vi "Create PID Controller.vi"(8 "error in (no error)":errorcluster, 10 "Settings":T3, 11 "Custom Device Ref":refnum<k24>) -> (0 "error out":errorcluster, 3 "Custom Device Ref":refnum<k24>)   [LabVIEW 2013, in "Control SysDef API.lvlib"]
uses:
  Control SysDef API.lvlib
  NationalInstruments.VeriStand.SystemDefinitionAPI
  Shared/Types/Controller Settings.ctl
  Shared/Types/PID Parameters.ctl
  Shared/Types/Action.ctl
  Shared/Constants.vi
  <vilib>/NI Veristand/Custom Device API/NI VeriStand - Set Item Property.vi
  <vilib>/NI Veristand/Custom Device API/Set Item Property (Double).vi
  <vilib>/NI Veristand/Custom Device API/Set Item Property (Boolean).vi
  <vilib>/NI Veristand/Custom Device Tools/Custom Device Utility Library/NI VeriStand - Search for Item.vi
  <vilib>/NI Veristand/Custom Device Tools/Custom Device Utility Library/NI VeriStand - Search for Item by GUID.vi
  <vilib>/NI Veristand/Custom Device API/NI VeriStand - Add Custom Device Channel.vi
  <vilib>/NI Veristand/Custom Device API/NI VeriStand - Remove Custom Device Item.vi
  <vilib>/NI Veristand/Custom Device API/Set Item Property (String).vi
  Shared/Control Addon Shared.lvlib
  <vilib>/NI Veristand/Custom Device API/Custom Device API.lvlib
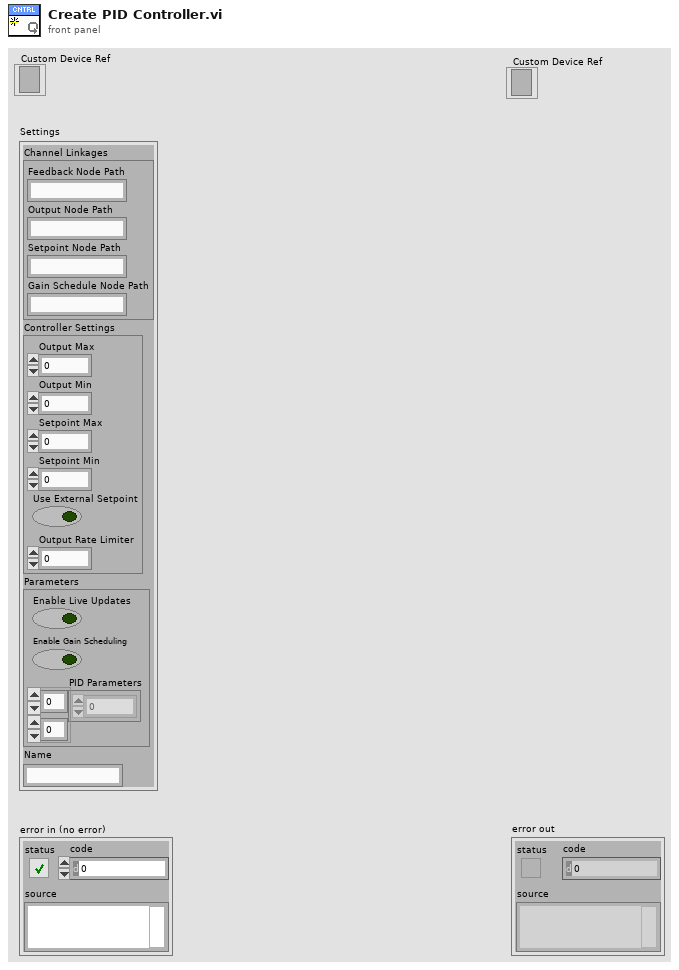
[diagram p1: front panel]
types:
  T1 = typedef "Control Addon Shared.lvlib/Controller Settings.ctl" = cluster{"Output Max":dbl, "Output Min":dbl, "Setpoint Max":dbl, "Setpoint Min":dbl, "Use External Setpoint":bool, "Output Rate Limiter":dbl}
  T2 = typedef "Control Addon Shared.lvlib/PID Parameters.ctl" = cluster{"Enable Live Updates":bool, "Enable Gain Scheduling":bool, "PID Parameters":dbl[][]}
  T3 = cluster{"Channel Linkages":cluster{"Feedback Node Path":string, "Output Node Path":string, "Setpoint Node Path":string, "Gain Schedule Node Path":string}, "Controller Settings":T1, "Parameters":T2, "Name":string}
  T4 = typedef "Control Addon Shared.lvlib/Action.ctl" = enum16{"Get", "Set"}
  T5 = typedef "Custom Device API.lvlib/Custom Device Item Ref.ctl" = u64
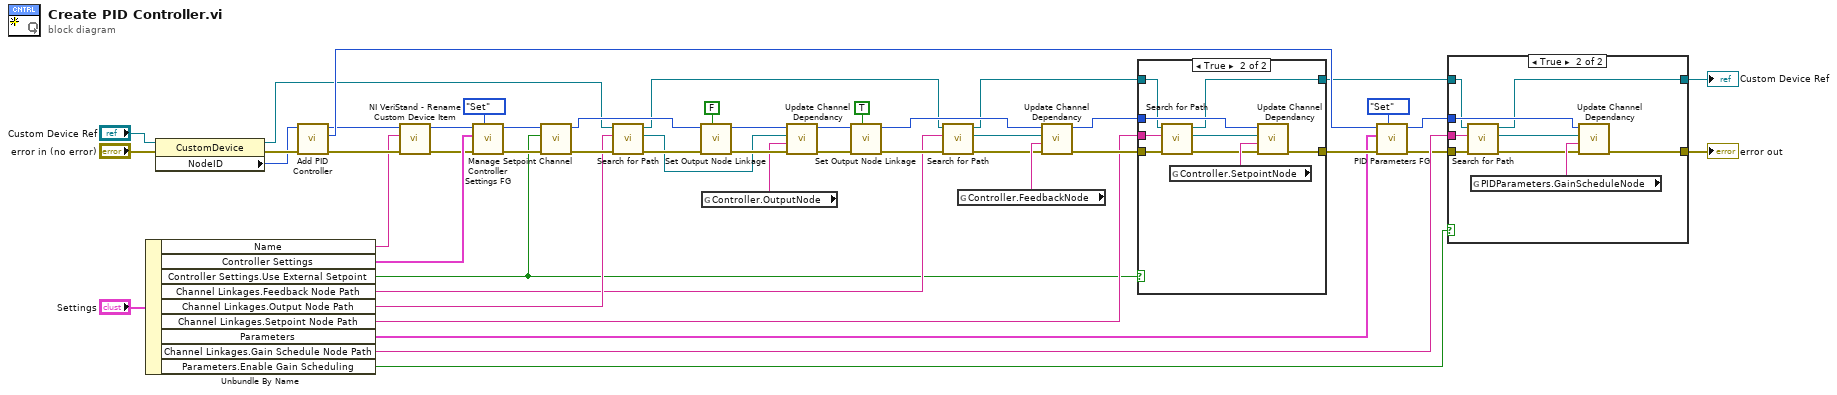
[diagram p0: block diagram]
diagram:
  n1 = Unbundle By Name("Settings") -> ("Name"=w3:string, "Controller Settings"=w27:T1, "Controller Settings.Use External Setpoint"=w8:bool, "Channel Linkages.Feedback Node Path"=w18:string, "Channel Linkages.Output Node Path"=w23:string, "Channel Linkages.Setpoint Node Path"=w15:string, "Parameters"=w2:T2, "Channel Linkages.Gain Schedule Node Path"=w14:string, "Parameters.Enable Gain Scheduling"=w10:bool)
  n2 = property class="CustomDevice"(reference="Custom Device Ref", error in="error in (no error)") -> (reference out=w24:refnum<k24>, error out=w48:errorcluster, "NodeID"=w38:u64)
  n3 = call "Add PID Controller.vi"("error in (no error)"=w48, "Node Ptr"=w38) -> ("error out"=w6:errorcluster, "Controller PID Parameters Ref"=w31:T5, "Controller Ref Out"=w7:T5)  [unwired: 7 in]
  n4 = call <vilib>:"NI VeriStand - Rename Custom Device Item.vi"("error in (no error)"=w6, "New Name"=w3, "Item Ref in"=w7) -> ("error out"=w5:errorcluster, "Item Ref out"=w4:T5)  [unwired: 6 in, 1 out]
  n5 = call "Controller Settings FG.vi"("Action"=Action."Set", "error in (no error)"=w5, "Controller Settings"=w27, "Node Ptr"=w4) -> ("error out"=w36:errorcluster, "Item Ref out"=w37:T5)  [unwired: 5 in, 1 out]
  n6 = call "Manage Setpoint Channel.vi"("error in (no error)"=w36, "Use External Setpoint"=w8, "Node Ptr"=w37) -> ("error out"=w26:errorcluster, "Node Ptr out"=w35:T5)  [unwired: 7 in]
  n7 = call "Search for Path.vi"("error in (no error)"=w26, "nodepath"=w23, "Custom Device Ref"=w24) -> ("error out"=w25:errorcluster, "BaseNodeType"=w22:refnum<k24>, "Custom Device Ref"=w19:refnum<k24>)  [unwired: 6 in]
  n8 = call "Set Output Node Linkage.vi"("Add?"=FALSE, "error in"=w25, "Section Ref in"=w35) -> ("error out"=w45:errorcluster, "Item Ref out"=w46:T5)  [unwired: 7 in]
  n9 = global read "Constants.vi" "Controller.OutputNode"() -> (w40:string)
  n10 = call "Update Channel Dependancy.vi"("error in (no error)"=w45, "NodeName"=w40, "Data"=w22, "Item Ref in"=w46) -> ("error out"=w41:errorcluster, "Item Ref out"=w42:T5)  [unwired: 6 in]
  n11 = call "Set Output Node Linkage.vi"("Add?"=TRUE, "error in"=w41, "Section Ref in"=w42) -> ("error out"=w21:errorcluster, "Item Ref out"=w34:T5)  [unwired: 7 in]
  n12 = call "Search for Path.vi"("error in (no error)"=w21, "nodepath"=w18, "Custom Device Ref"=w19) -> ("error out"=w20:errorcluster, "BaseNodeType"=w17:refnum<k24>, "Custom Device Ref"=w9:refnum<k24>)  [unwired: 6 in]
  n13 = global read "Constants.vi" "Controller.FeedbackNode"() -> (w39:string)
  n14 = call "Update Channel Dependancy.vi"("error in (no error)"=w20, "NodeName"=w39, "Data"=w17, "Item Ref in"=w34) -> ("error out"=w16:errorcluster, "Item Ref out"=w33:T5)  [unwired: 6 in]
  n15 = case shown="True" w8 {
    tunnel: w33 -> [_ w60]
    tunnel: w9 -> [w52 w59]
    tunnel: w16 -> [w51 w58]
    tunnel: w15 -> [_ w55]
    tunnel: [w51 w54] -> w13
    tunnel: [w52 w53] -> w11
    frame False {
    }
    frame True {
      n16 = call "Search for Path.vi"("error in (no error)"=w58, "nodepath"=w55, "Custom Device Ref"=w59) -> ("error out"=w57:errorcluster, "BaseNodeType"=w56:refnum<k24>, "Custom Device Ref"=w53:refnum<k24>)  [unwired: 6 in]
      n17 = global read "Constants.vi" "Controller.SetpointNode"() -> (w61:string)
      n18 = call "Update Channel Dependancy.vi"("error in (no error)"=w57, "NodeName"=w61, "Data"=w56, "Item Ref in"=w60) -> ("error out"=w54:errorcluster)  [unwired: 6 in, 1 out]
    }
  }
  n19 = call "PID Parameters FG.vi"("Action"=Action."Set", "error in (no error)"=w13, "Parameters"=w2, "Node Ptr"=w31) -> ("error out"=w12:errorcluster, "Item Ref out"=w29:T5)  [unwired: 5 in, 1 out]
  n20 = case shown="True" w10 {
    tunnel: [w63 w71] -> w30
    tunnel: w29 -> [_ w70]
    tunnel: w14 -> [_ w69]
    tunnel: w12 -> [w63 w68]
    tunnel: w11 -> [w62 w67]
    tunnel: [w62 w64] -> w1
    frame False {
    }
    frame True {
      n21 = call "Search for Path.vi"("error in (no error)"=w68, "nodepath"=w69, "Custom Device Ref"=w67) -> ("error out"=w65:errorcluster, "BaseNodeType"=w66:refnum<k24>, "Custom Device Ref"=w64:refnum<k24>)  [unwired: 6 in]
      n22 = global read "Constants.vi" "PIDParameters.GainScheduleNode"() -> (w72:string)
      n23 = call "Update Channel Dependancy.vi"("error in (no error)"=w65, "NodeName"=w72, "Data"=w66, "Item Ref in"=w70) -> ("error out"=w71:errorcluster)  [unwired: 6 in, 1 out]
    }
  }
  "Custom Device Ref" <- w1
  "error out" <- w30
